vi "ge_GetHdrInfo.vi"(7 "ge_DAQManDefinitions":T1, 11 "MeasType":T4) -> (1 "Glbl Ctrls":T2[](array[typedef]), 2 "Hdr Widths":i32[](array[numeric]), 3 "Hdr Name":T3[](array[typedef]))   [LabVIEW 2018]
uses:
  Custom Ctrls/ge_MeasType.ctl
  Common/Controls/HeaderNames.ctl
  Custom Ctls Table/ge_GlblCtrls.ctl
  Common/Controls/DAQMan Definitions.ctl
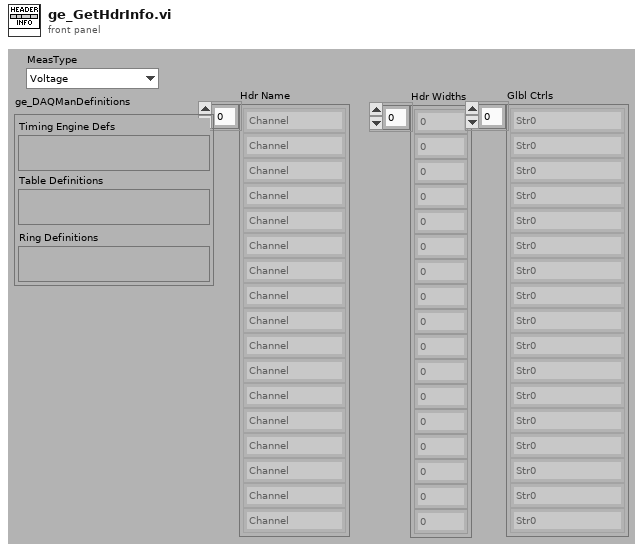
[diagram p1: front panel]
types:
  T1 = typedef "DAQMan Definitions.ctl" = cluster{"Timing Engine Defs":variant, "Table Definitions":variant, "Ring Definitions":variant}
  T2 = typedef "ge_GlblCtrls.ctl" = enum16{"Str0", "Bool0", "Bool1", "Int0", "Ring0", "Ring1", "Ring2", "Ring3", "Dbl0", "Dbl1", "Dbl2", "Dbl3", "Cal0", "Cal1", "Cal2", "None"}
  T3 = typedef "HeaderNames.ctl" = enum16{"Channel", "Device", "Spacer", "Description", "MB", "Range", "Terminal", "Coupling", "Thresh (V)", "Pulse/Rev", "Slope", "Min EU", "Min RPM", "mV/EU", "Iex", "Temp Units", "Type", "CJC Src", "CJC Val", "Ro", "Wire Cfg", "Strain Mode", "Vex", "Bridge Type", "GF", "Gauge Res", "Poisson", "Lead Res", "Init Strain", "GAF", "Scale", "Offset", "Unit (EU)", "dB?", "dB Ref", "Cal Mag", "Cal Units", "Max Temp", "Min Temp", "Max Strain", "Min Strain"}
  T4 = typedef "ge_MeasType.ctl" = enum16{"Voltage", "Frequency", "Tachometer", "Dynamic", "Thermocouple", "RTD", "Strain", "Current", "Resistance"}
  T5 = typedef "ge_ColDef.ctl" = cluster{"ge_HdrNames":T3, "HdrInfo":T6}
  T6 = typedef "ge_HdrInfo.ctl" = cluster{"Hdr Width":i32, "Glbl Ctrl":T2}
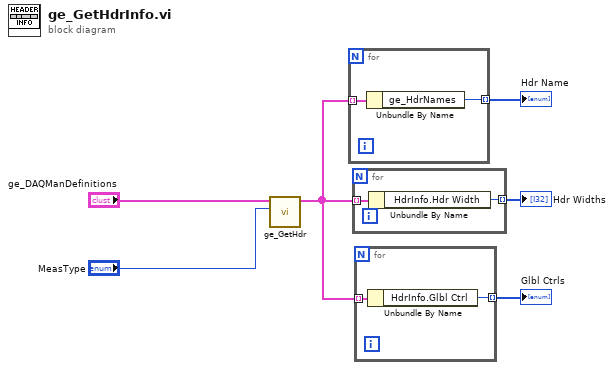
[diagram p0: block diagram]
diagram:
  n1 = call "ge_GetHdr.vi"("MeasType"="MeasType", "ge_DAQManDefinitions"="ge_DAQManDefinitions") -> ("Table Hdrs"=w4:T5[])  [unwired: 8 in, 1 out]
  n2 = for {
    tunnel: w4 -> [w8] mode=indexing
    tunnel: [w7] -> w2 mode=indexing
    n3 = Unbundle By Name(w8) -> ("ge_HdrNames"=w7:T3)
  }
  "Hdr Name" <- w2
  n4 = for {
    tunnel: w4 -> [w10] mode=indexing
    tunnel: [w9] -> w6 mode=indexing
    n5 = Unbundle By Name(w10) -> ("HdrInfo.Hdr Width"=w9:i32)
  }
  "Hdr Widths" <- w6
  n6 = for {
    tunnel: w4 -> [w12] mode=indexing
    tunnel: [w11] -> w1 mode=indexing
    n7 = Unbundle By Name(w12) -> ("HdrInfo.Glbl Ctrl"=w11:T2)
  }
  "Glbl Ctrls" <- w1
